vi "standardButtons.vi"(8 "Error In":errorcluster, 11 "QMessageBox In":refnum<class "QMessageBox.lvclass">) -> (0 "Error Out":errorcluster, 2 "Value":T1 items=["NoButton"=0, "Ok"=1024, "Save"=2048, "SaveAll"=4096, "Open"=8192, "Yes"=16384, "YesToAll"=32768, "No"=65536, "NoToAll"=131072, "Abort"=262144, "Retry"=524288, "Ignore"=1048576, "Close"=2097152, "Cancel"=4194304, "Discard"=8388608, "Help"=16777216, "Apply"=33554432, "Reset"=67108864, "RestoreDefaults"=134217728], 3 "QMessageBox Out":refnum<class "QMessageBox.lvclass">)   [LabVIEW 2014, in "QMessageBox.lvclass"]
doc: "LabVIEW-specific documentation is not yet available. See <b>https://doc.qt.io/qt-5/qmessagebox.html#standardButtons</b>"
uses:
  QMessageBox.lvclass
  StandardButton.ctl
  LQ Core/LQIdentity/LQIdentity.lvclass/LQIdentity.ctl
  LQ Core/LQ Core.lvlib
  LQ Core/LQIdentity/LQIdentity.lvclass
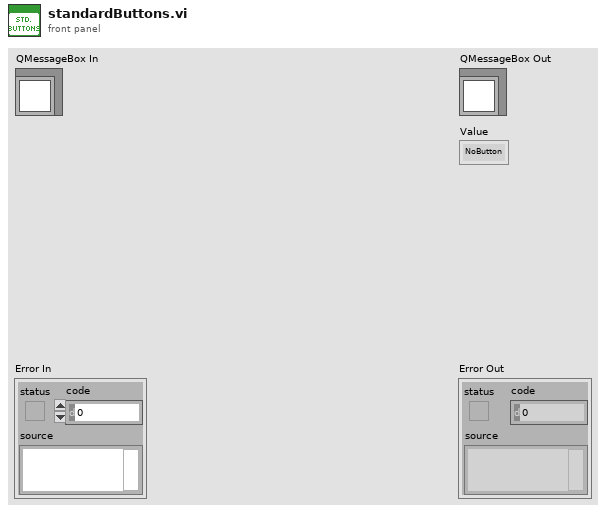
[diagram p1: front panel]
types:
  T1 = typedef "QMessageBox.lvclass/StandardButton.ctl" = i32
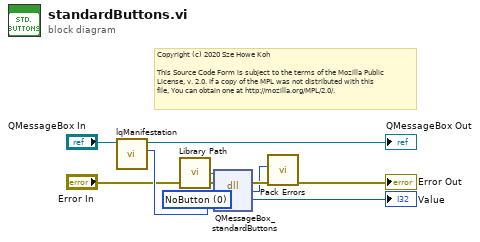
[diagram p0: block diagram]
diagram:
  w7 = T1 0 items=["NoButton"=0, "Ok"=1024, "Save"=2048, "SaveAll"=4096, "Open"=8192, "Yes"=16384, "YesToAll"=32768, "No"=65536, "NoToAll"=131072, "Abort"=262144, "Retry"=524288, "Ignore"=1048576, "Close"=2097152, "Cancel"=4194304, "Discard"=8388608, "Help"=16777216, "Apply"=33554432, "Reset"=67108864, "RestoreDefaults"=134217728] ("retVal")
  # "Copyright (c) 2020 Sze Howe Koh\n\nThis Source Code Form is subject to the terms of the Mozilla Public\nLicense, v. 2.0. If a copy of the MPL was not distributed with this\nfile, You can obtain one at http://mozilla.org/MPL/2.0/."
  n1 = call "lqManifestation.vi"("LQIdentity in"="QMessageBox In") -> ("Manifestation"=w5:u64, "LQIdentity out"=→"QMessageBox Out":refnum<class "QMessageBox.lvclass">)  [unwired: 9 in]
  n2 = call "Library Path.vi"() -> ("Library Path"=w6:path)
  n3 = dll-call lib="?" fn="QMessageBox_standardButtons"(path in=w6, error in="Error In", "_retVal"=w7, "_instance"=w5) -> (error out=w3:errorcluster, w1:i32, "_retVal"=→"Value":i32)  [unwired: 2 in, 1 out]
  n4 = call "Pack Errors.vi"("Error In"=w3, "Error Code"=w1) -> ("Error Out"=→"Error Out":errorcluster)  [unwired: 9 in]
